vi "dB.vi"(1 "V":dbl) -> (0 "dB":dbl)   [LabVIEW 2013]
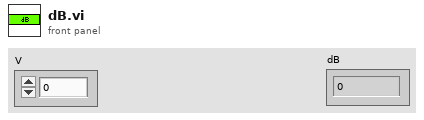
[diagram p1: front panel]
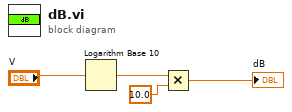
[diagram p0: block diagram]
diagram:
  n1 = Logarithm Base 10(1:"V") -> (0:w3:dbl)
  n2 = Multiply(x=w3, y=10.0) -> (x*y=→"dB":dbl)
